vi "Imaging_Lick.vi"() -> ()   [LabVIEW 2010]
panel:
  out "シャッター":bool
  out "Hit回数":i32
  out "Hit率":dbl format="%#_2f"
  in  "報酬回数":i32=2
  out "Cue間隔":i32
  out "CR回数":i32
  out "B回数":i32
  out "CR配列":dbl[](array[numeric])
  out "計算回数":i32=20
  out "Lick終了時刻":i32
  out "Cue開始時刻":i32
  out "延長時間":i32=1000
  in  "終了回数":i32=5
  out "連続Miss":i32
  out "Trial回数":i32
  out "CR率":dbl format="%#_2f"
  out "開始時刻":i32
  out "Lick判定":i32
  out "Cue間隔2":i32=10500
  out "Cue間隔1":i32=6000
  out "Ans時間":i32=1000
  in  "Cue B":bool
  out "Cue判定":i32
  out "乱数":dbl
  out "Cue時間":i32=500
  out "経過時間(s)":i32
  out "総報酬回数":i32
  in  "保存":bool=TRUE
  in  "No.":i32=1
  in  "マウス名":string="M07"
  out "保存ファイル名":path
  in  "Cue A":bool
  out "レート(Hz)":dbl=200.0
  out "サンプル数":i32=1
  out "現在時刻":i32
  in  "stop (F)":bool caption="停止(F)"
  out "波形チャート":dynamicdata(graph)
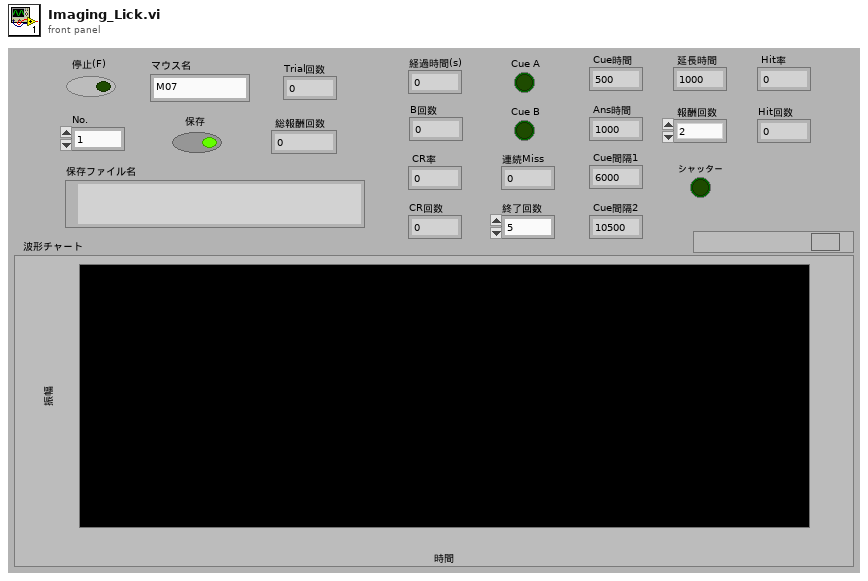
[diagram p1: front panel]
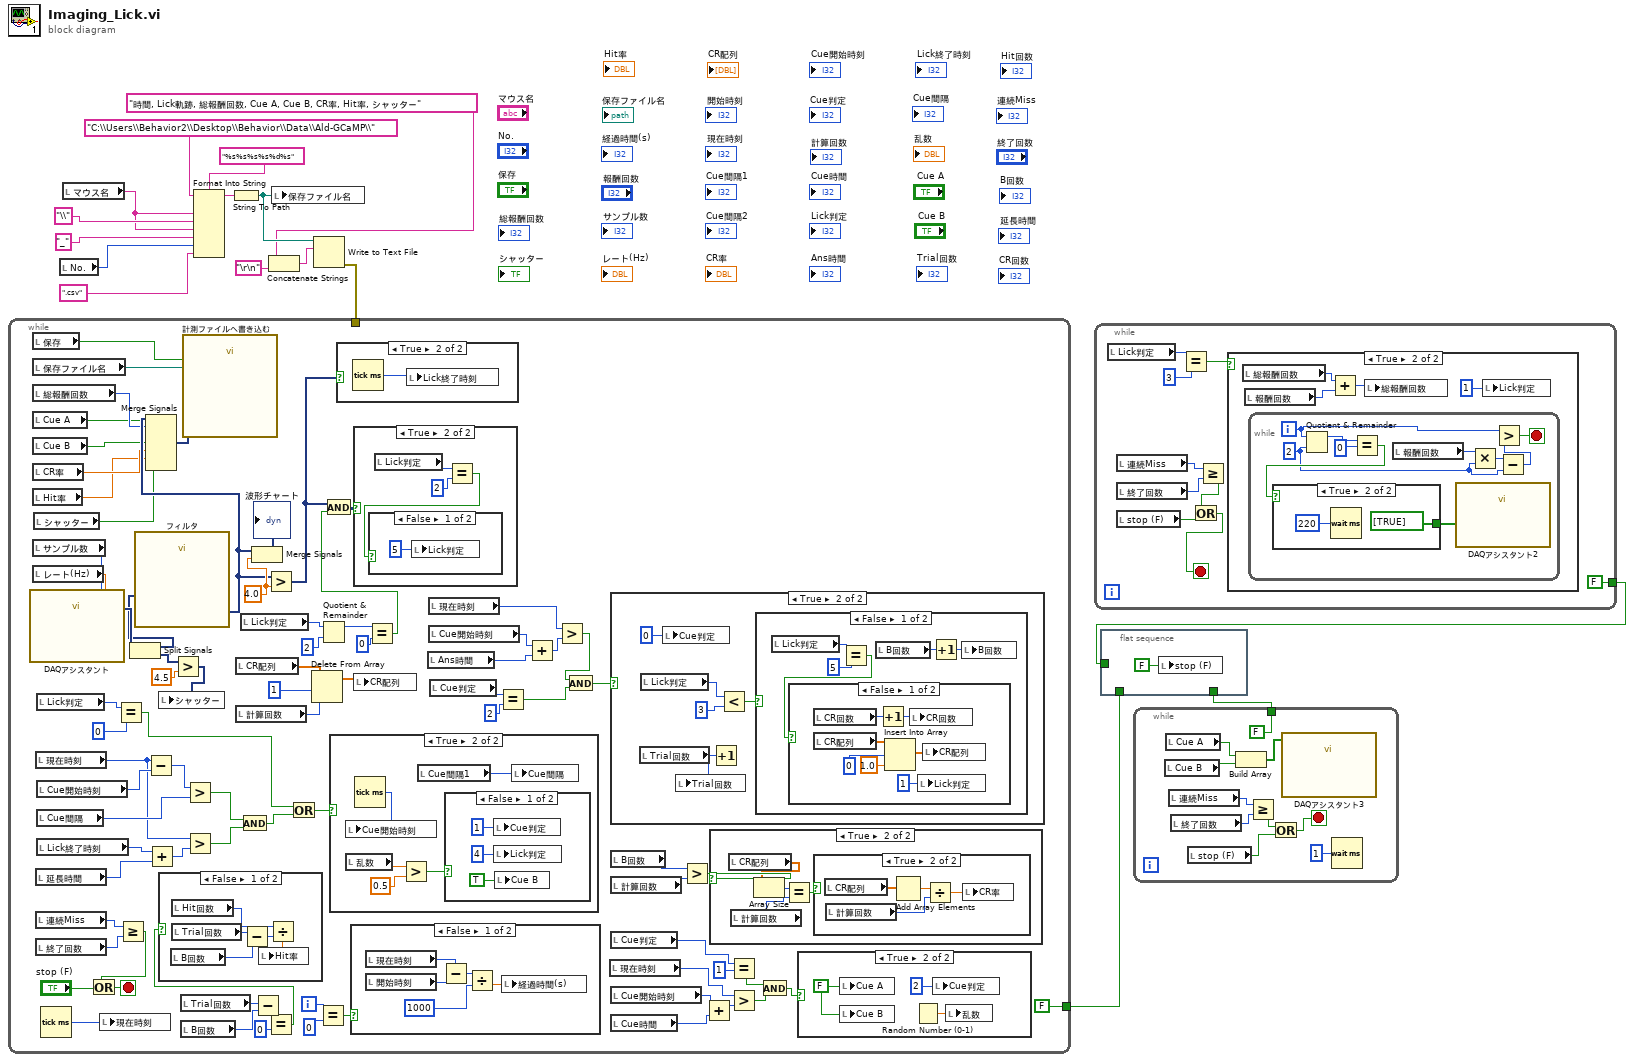
[diagram p0: block diagram]
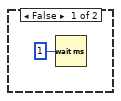
[diagram p2: hidden frame]
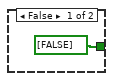
[diagram p3: hidden frame]
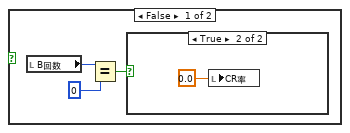
[diagram p5: hidden frame]
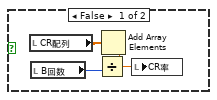
[diagram p6: hidden frame]
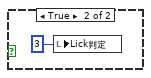
[diagram p9: hidden frame]
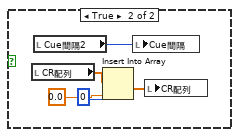
[diagram p12: hidden frame]
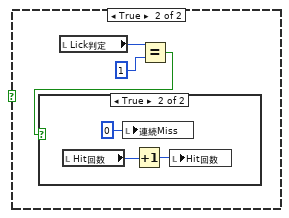
[diagram p13: hidden frame]
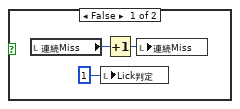
[diagram p14: hidden frame]
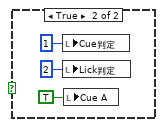
[diagram p17: hidden frame]
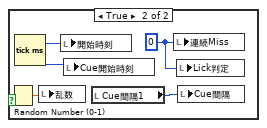
[diagram p18: hidden frame]
diagram:
  n1 = local read "No."() -> (w5:i32)
  n2 = local read "マウス名"() -> (w7:string)
  n3 = Format Into String(format string="%s%s%s%s%d%s" ("形式文字列"), initial string="C:\\Users\\Behavior2\\Desktop\\Behavior\\Data\\Ald-GCaMP\\" ("初期文字列"), w7, "\\" ("入力 4"), w7, "_" ("入力 4"), w5, ".csv" ("入力 9")) -> (resulting string=w16:string)  [unwired: 1 in, 1 out]
  n4 = String To Path(string=w16) -> (path=w12:path)
  n5 = Concatenate Strings("時間, Lick軌跡, 総報酬回数, Cue A, Cue B, CR率, Hit率, シャッター" ("文字列"), "\r\n") -> (w15:string)
  n6 = local write "保存ファイル名"(w12) -> ()
  n7 = Write to Text File(file (use dialog)=w12, text=w15) -> (error out=w11:errorcluster)  [unwired: 2 in, 2 out]
  n8 = while {
    tunnel: w11 -> [_]
    tunnel: [FALSE] -> w2
    i -> [w89]
    stop <- w76 stop-if-true
    w88 = 4.0 ("y")
    n9 = local read "保存"() -> (w93:bool)
    n10 = local read "保存ファイル名"() -> (w87:path)
    n11 = local read "総報酬回数"() -> (w85:i32)
    n12 = local read "Cue A"() -> (w72:bool)
    n13 = local read "Cue B"() -> (w71:bool)
    n14 = local read "CR率"() -> (w70:dbl)
    n15 = local read "Hit率"() -> (w30:dbl)
    n16 = local read "サンプル数"() -> (w95:i32)
    n17 = local read "レート(Hz)"() -> (w94:dbl)
    n18 = call "DAQアシスタント"("レート"=w94, "サンプル数"=w95) -> ("data"=w20:dynamicdata)  [unwired: 14 in, 3 out]
    n19 = local read "シャッター"() -> (w21:bool)
    n20 = local read "現在時刻"() -> (w35:i32)
    n21 = local read "延長時間"() -> (w37:i32)
    n22 = local read "連続Miss"() -> (w74:i32)
    n23 = local read "終了回数"() -> (w73:i32)
    n24 = local read "Lick判定"() -> (w44:i32)
    n25 = local read "Cue開始時刻"() -> (w41:i32)
    n26 = local read "Cue間隔"() -> (w39:i32)
    n27 = local read "Lick終了時刻"() -> (w38:i32)
    n28 = Tick Count (ms)() -> (millisecond timer value=w96:u32)
    n29 = local write "現在時刻"(w96) -> ()
    n30 = Equal?(x=w44, y=0) -> (x = y?=w32:bool)
    n31 = Greater Or Equal?(x=w74, y=w73) -> (x >= y?=w75:bool)
    n32 = Or(x=w75, y="stop (F)") -> (x .or. y?=w76:bool)
    n33 = Split Signals(w20) -> (w19:dynamicdata, w18:dynamicdata)  [unwired: 2 in]
    n34 = call "フィルタ"("Signal"=w19) -> ("Filtered Signal"=w86:dynamicdata)  [unwired: 9 in, 1 out]
    n35 = Merge Signals(w86, w85, w72, w71, w70, w30, w21) -> (w91:dynamicdata)
    n36 = Subtract(x=w35, y=w41) -> (x-y=w40:i32)
    n37 = Add(x=w38, y=w37) -> (x+y=w36:i32)
    n38 = Greater?(x=w18, y=4.5) -> (0:w22:dynamicdata)
    n39 = local write "シャッター"(w22) -> ()
    n40 = local read "Trial回数"() -> (w28:i32)
    n41 = local read "B回数"() -> (w27:i32)
    n42 = call "計測ファイルへ書き込む"("Signals"=w91, "Enable"=w93, "Filename"=w87) -> ()  [unwired: 14 in, 3 out]
    n43 = Greater?(x=w40, y=w39) -> (0:w34:bool)
    n44 = Greater?(x=w35, y=w36) -> (0:w33:bool)
    n45 = local read "CR配列"() -> (w58:dbl[])
    n46 = local read "計算回数"() -> (w56:i32)
    n47 = And(x=w34, y=w33) -> (x .and. y?=w31:bool)
    n48 = local read "Lick判定"() -> (w51:i32)
    n49 = Merge Signals(w86, w88) -> (→"波形チャート":dynamicdata)
    n50 = Subtract(x=w28, y=w27) -> (x-y=w26:i32)
    n51 = Greater?(x=w86, y=w88) -> (0:w67:dynamicdata)
    n52 = Equal?(x=w26, y=0) -> (x = y?=w25:bool)
    n53 = case shown="FALSE" w25 {
      frame False {
        n54 = local read "B回数"() -> (w100:i32)
        n55 = local read "Hit回数"() -> (w98:i32)
        n56 = local read "Trial回数"() -> (w101:i32)
        n57 = Subtract(x=w101, y=w100) -> (x-y=w99:i32)
        n58 = Divide(x=w98, y=w99) -> (x/y=w97:dbl)
        n59 = local write "Hit率"(w97) -> ()
      }
      frame True {
      }
    }
    n60 = Or(x=w32, y=w31) -> (x .or. y?=w42:bool)
    n61 = Delete From Array(array=w58, length=1 ("長さ"), index=w56) -> (array with subset deleted=w57:dbl[])  [unwired: 1 out]
    n62 = Equal?(x=w89, y=0) -> (x = y?=w90:bool)
    n63 = Quotient & Remainder(x=w51, y=2) -> (x-y*floor(x/y)=w49:i32)  [unwired: 1 out]
    n64 = case shown="TRUE" w42 {
      frame False {
      }
      frame True {
        n65 = local read "乱数"() -> (w163:dbl)
        n66 = Tick Count (ms)() -> (millisecond timer value=w160:u32)
        n67 = local write "Cue開始時刻"(w160) -> ()
        n68 = Greater?(x=w163, y=0.5) -> (0:w162:bool)
        n69 = local read "Cue間隔1"() -> (w159:i32)
        n70 = case shown="FALSE" w162 {
          frame False {
            n71 = local write "Cue判定"(1 ("Cue判定")) -> ()
            n72 = local write "Lick判定"(4 ("Lick判定")) -> ()
            n73 = local write "Cue B"(TRUE ("Cue B")) -> ()
          }
          frame True {
            n74 = local write "Cue判定"(1 ("Cue判定")) -> ()
            n75 = local write "Lick判定"(2 ("Lick判定")) -> ()
            n76 = local write "Cue A"(TRUE ("Cue A")) -> ()
          }
        }
        n77 = local write "Cue間隔"(w159) -> ()
      }
    }
    n78 = case shown="TRUE" w67 {
      frame False {
      }
      frame True {
        n79 = Tick Count (ms)() -> (millisecond timer value=w123:u32)
        n80 = local write "Lick終了時刻"(w123) -> ()
      }
    }
    n81 = case shown="FALSE" w90 {
      frame False {
        n82 = local read "現在時刻"() -> (w171:i32)
        n83 = local read "開始時刻"() -> (w173:i32)
        n84 = Subtract(x=w171, y=w173) -> (x-y=w172:i32)
        n85 = Divide(x=w172, y=1000) -> (x/y=w170:dbl)
        n86 = local write "経過時間(s)"(w170) -> ()
      }
      frame True {
        w176 = 0 ("Trial回数")
        n87 = Random Number (0-1)() -> (number: 0 to 1=w178:dbl)
        n88 = Tick Count (ms)() -> (millisecond timer value=w177:u32)
        n89 = local write "乱数"(w178) -> ()
        n90 = local write "開始時刻"(w177) -> ()
        n91 = local write "Cue開始時刻"(w177) -> ()
        n92 = local read "Cue間隔1"() -> (w175:i32)
        n93 = local write "連続Miss"(w176) -> ()
        n94 = local write "Lick判定"(w176) -> ()
        n95 = local write "Cue間隔"(w175) -> ()
      }
    }
    n96 = local write "CR配列"(w57) -> ()
    n97 = Equal?(x=w49, y=0) -> (x = y?=w45:bool)
    n98 = And(x=w67, y=w45) -> (x .and. y?=w64:dynamicdata)
    n99 = case shown="TRUE" w64 {
      frame False {
      }
      frame True {
        n100 = local read "Lick判定"() -> (w120:i32)
        n101 = Equal?(x=w120, y=2) -> (x = y?=w118:bool)
        n102 = case shown="FALSE" w118 {
          frame False {
            n103 = local write "Lick判定"(5 ("Lick判定")) -> ()
          }
          frame True {
            n104 = local write "Lick判定"(3 ("Lick判定")) -> ()
          }
        }
      }
    }
    n105 = local read "Ans時間"() -> (w65:i32)
    n106 = local read "現在時刻"() -> (w48:i32)
    n107 = local read "Cue開始時刻"() -> (w66:i32)
    n108 = local read "Cue判定"() -> (w63:i32)
    n109 = Equal?(x=w63, y=2) -> (x = y?=w62:bool)
    n110 = Add(x=w66, y=w65) -> (x+y=w47:i32)
    n111 = Greater?(x=w48, y=w47) -> (0:w46:bool)
    n112 = And(x=w46, y=w62) -> (x .and. y?=w60:bool)
    n113 = local read "現在時刻"() -> (w80:i32)
    n114 = case shown="TRUE" w60 {
      frame False {
      }
      frame True {
        n115 = local read "Trial回数"() -> (w128:i32)
        n116 = local read "Lick判定"() -> (w125:i32)
        n117 = local write "Cue判定"(0 ("Cue判定")) -> ()
        n118 = Increment(x=w128) -> (x+1=w129:i32)
        n119 = local write "Trial回数"(w129) -> ()
        n120 = Less?(x=w125, y=3) -> (x < y?=w126:bool)
        n121 = case shown="FALSE" w126 {
          frame False {
            n122 = local read "Lick判定"() -> (w134:i32)
            n123 = Equal?(x=w134, y=5) -> (x = y?=w132:bool)
            n124 = case shown="FALSE" w132 {
              frame False {
                n125 = local read "CR回数"() -> (w137:i32)
                n126 = local read "CR配列"() -> (w138:dbl[])
                n127 = Increment(x=w137) -> (x+1=w136:i32)
                n128 = Insert Into Array(array=w138, index=0 ("指標"), new element=1.0 ("新規要素/部分配列")) -> (w139:dbl[])
                n129 = local write "CR回数"(w136) -> ()
                n130 = local write "Lick判定"(1 ("Lick判定")) -> ()
                n131 = local write "CR配列"(w139) -> ()
              }
              frame True {
                n132 = local read "CR配列"() -> (w143:dbl[])
                n133 = local read "Cue間隔2"() -> (w142:i32)
                n134 = Insert Into Array(array=w143, index=0 ("指標"), new element=0.0 ("新規要素/部分配列")) -> (w146:dbl[])
                n135 = local write "Cue間隔"(w142) -> ()
                n136 = local write "CR配列"(w146) -> ()
              }
            }
            n137 = local read "B回数"() -> (w131:i32)
            n138 = Increment(x=w131) -> (x+1=w130:i32)
            n139 = local write "B回数"(w130) -> ()
          }
          frame True {
            n140 = local read "Lick判定"() -> (w149:i32)
            n141 = Equal?(x=w149, y=1) -> (x = y?=w147:bool)
            n142 = case shown="TRUE" w147 {
              frame False {
                n143 = local read "連続Miss"() -> (w152:i32)
                n144 = local write "Lick判定"(1 ("Lick判定")) -> ()
                n145 = Increment(x=w152) -> (x+1=w151:i32)
                n146 = local write "連続Miss"(w151) -> ()
              }
              frame True {
                n147 = local read "Hit回数"() -> (w154:i32)
                n148 = local write "連続Miss"(0 ("連続Miss")) -> ()
                n149 = Increment(x=w154) -> (x+1=w153:i32)
                n150 = local write "Hit回数"(w153) -> ()
              }
            }
          }
        }
      }
    }
    n151 = local read "B回数"() -> (w55:i32)
    n152 = local read "計算回数"() -> (w54:i32)
    n153 = local read "Cue判定"() -> (w84:i32)
    n154 = local read "Cue開始時刻"() -> (w69:i32)
    n155 = local read "Cue時間"() -> (w78:i32)
    n156 = Greater?(x=w55, y=w54) -> (0:w53:bool)
    n157 = Add(x=w69, y=w78) -> (x+y=w68:i32)
    n158 = case shown="TRUE" w53 {
      frame False {
        n159 = local read "B回数"() -> (w104:i32)
        n160 = Equal?(x=w104, y=0) -> (x = y?=w102:bool)
        n161 = case shown="TRUE" w102 {
          frame False {
            n162 = local read "CR配列"() -> (w106:dbl[])
            n163 = local read "B回数"() -> (w108:i32)
            n164 = Add Array Elements(numeric array=w106) -> (sum=w105:dbl)
            n165 = Divide(x=w105, y=w108) -> (x/y=w107:dbl)
            n166 = local write "CR率"(w107) -> ()
          }
          frame True {
            n167 = local write "CR率"(0.0 ("正解率")) -> ()
          }
        }
      }
      frame True {
        n168 = local read "CR配列"() -> (w111:dbl[])
        n169 = local read "計算回数"() -> (w110:i32)
        n170 = Array Size(array=w111) -> (size(s)=w113:i32)
        n171 = Equal?(x=w113, y=w110) -> (x = y?=w112:bool)
        n172 = case shown="TRUE" w112 {
          frame False {
          }
          frame True {
            n173 = local read "CR配列"() -> (w115:dbl[])
            n174 = local read "計算回数"() -> (w117:i32)
            n175 = Add Array Elements(numeric array=w115) -> (sum=w114:dbl)
            n176 = Divide(x=w114, y=w117) -> (x/y=w116:dbl)
            n177 = local write "CR率"(w116) -> ()
          }
        }
      }
    }
    n178 = Equal?(x=w84, y=1) -> (x = y?=w82:bool)
    n179 = Greater?(x=w80, y=w68) -> (0:w79:bool)
    n180 = And(x=w82, y=w79) -> (x .and. y?=w81:bool)
    n181 = case shown="TRUE" w81 {
      frame False {
      }
      frame True {
        w156 = FALSE ("Cue A")
        n182 = local write "Cue A"(w156) -> ()
        n183 = local write "Cue B"(w156) -> ()
        n184 = Random Number (0-1)() -> (number: 0 to 1=w158:dbl)
        n185 = local write "Cue判定"(2 ("Cue判定")) -> ()
        n186 = local write "乱数"(w158) -> ()
      }
    }
  }
  n187 = while {
    tunnel: [FALSE] -> w3
    stop <- w180 stop-if-true
    n188 = local read "Lick判定"() -> (w186:i32)
    n189 = local read "連続Miss"() -> (w184:i32)
    n190 = local read "終了回数"() -> (w183:i32)
    n191 = local read "stop (F)"() -> (w181:bool)
    n192 = Equal?(x=w186, y=3) -> (x = y?=w185:bool)
    n193 = Greater Or Equal?(x=w184, y=w183) -> (x >= y?=w182:bool)
    n194 = Or(x=w182, y=w181) -> (x .or. y?=w180:bool)
    n195 = case shown="TRUE" w185 {
      frame False {
        n196 = Wait (ms)(milliseconds to wait=u32 1 ("ミリ秒待機時間")) -> ()  [unwired: 1 out]
      }
      frame True {
        n197 = local read "総報酬回数"() -> (w191:i32)
        n198 = local read "報酬回数"() -> (w189:i32)
        n199 = while {
          i -> [w200]
          stop <- w197 stop-if-true
          w195 = 2 ("y")
          n200 = Quotient & Remainder(x=w200, y=w195) -> (x-y*floor(x/y)=w202:i32)  [unwired: 1 out]
          n201 = Equal?(x=w202, y=0) -> (x = y?=w199:bool)
          n202 = case shown="TRUE" w199 {
            tunnel: [bool[] [FALSE] ("data") bool[] [TRUE] ("data")] -> w198
            frame False {
            }
            frame True {
              n203 = Wait (ms)(milliseconds to wait=u32 220 ("ミリ秒待機時間")) -> ()  [unwired: 1 out]
            }
          }
          n204 = local read "報酬回数"() -> (w193:i32)
          n205 = call "DAQアシスタント2"("data"=w198) -> ()  [unwired: 17 in, 2 out]
          n206 = Multiply(x=w193, y=w195) -> (x*y=w196:i32)
          n207 = Subtract(x=w196, y=w195) -> (x-y=w194:i32)
          n208 = Greater?(x=w200, y=w194) -> (0:w197:bool)
        }
        n209 = Add(x=w191, y=w189) -> (x+y=w190:i32)
        n210 = local write "総報酬回数"(w190) -> ()
        n211 = local write "Lick判定"(1 ("Lick判定")) -> ()
      }
    }
  }
  n212 = flat-sequence {
    tunnel: w3 -> [_]
    tunnel: w2 -> [_]
    tunnel: w1 -> [_]
    frame #0 {
      n213 = local write "stop (F)"(FALSE ("stop (F)")) -> ()
    }
  }
  n214 = while {
    tunnel: [FALSE] -> w1
    stop <- w207 stop-if-true
    n215 = local read "Cue B"() -> (w215:bool)
    n216 = local read "Cue A"() -> (w216:bool)
    n217 = local read "連続Miss"() -> (w211:i32)
    n218 = local read "終了回数"() -> (w210:i32)
    n219 = local read "stop (F)"() -> (w208:bool)
    n220 = Build Array(w216, w215) -> (w214:bool[])
    n221 = Greater Or Equal?(x=w211, y=w210) -> (x >= y?=w209:bool)
    n222 = Or(x=w209, y=w208) -> (x .or. y?=w207:bool)
    n223 = call "DAQアシスタント3"("data"=w214) -> ()  [unwired: 17 in, 2 out]
    n224 = Wait (ms)(milliseconds to wait=u32 1 ("ミリ秒待機時間")) -> ()  [unwired: 1 out]
  }
